vi "CoordinateConvert_WorldCartesianToShoulderOriginCartesian_Array.vi"(1 "ArmPositionIn":T1[](array[typedef]), 2 "RobotDimensions":T2) -> (0 "ArmPositionRelativeToShoulder":T1[](array[typedef]))   [LabVIEW 2018]
uses:
  TypeDefs/ConfigComponents/Config_Dimensions.ctl
  TypeDefs/ArmAbsolutePosition.ctl
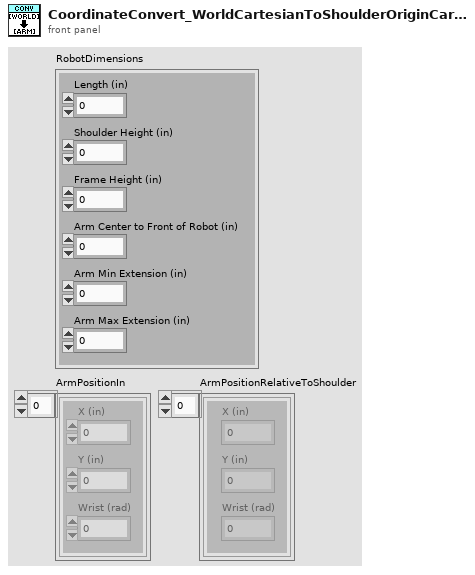
[diagram p1: front panel]
types:
  T1 = typedef "ArmAbsolutePosition.ctl" = cluster{"X (in)":dbl, "Y (in)":dbl, "Wrist (rad)":dbl}
  T2 = typedef "Config_Dimensions.ctl" = cluster{"Length (in)":dbl, "Shoulder Height (in)":dbl, "Frame Height (in)":dbl, "Arm Center to Front of Robot (in)":dbl, "Arm Min Extension (in)":dbl, "Arm Max Extension (in)":dbl}
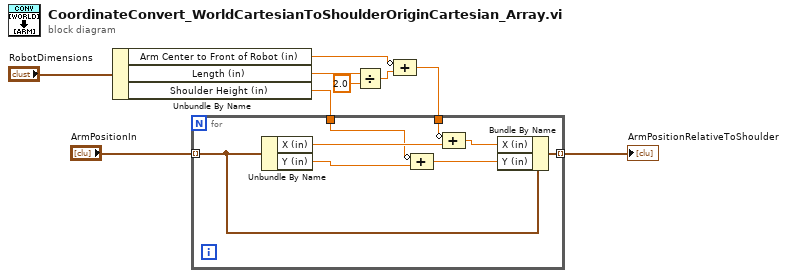
[diagram p0: block diagram]
diagram:
  n1 = Unbundle By Name("RobotDimensions") -> ("Arm Center to Front of Robot (in)"=w6:dbl, "Length (in)"=w8:dbl, "Shoulder Height (in)"=w4:dbl)
  n2 = Divide(x=w8, y=2.0) -> (x/y=w5:dbl)
  n3 = Compound Arithmetic op=ADD(invert w6, w5) -> (w3:dbl)
  n4 = for {
    tunnel: w4 -> [w10]
    tunnel: w3 -> [w16]
    tunnel: "ArmPositionIn" -> [w13] mode=indexing
    tunnel: [w12] -> w1 mode=indexing
    n5 = Unbundle By Name(w13) -> ("X (in)"=w15:dbl, "Y (in)"=w11:dbl)
    n6 = Compound Arithmetic op=ADD(invert w10, w11) -> (w17:dbl)
    n7 = Compound Arithmetic op=ADD(invert w16, w15) -> (w14:dbl)
    n8 = Bundle By Name(cluster=w13, "X (in)"=w14, "Y (in)"=w17) -> (w12:T1)
  }
  "ArmPositionRelativeToShoulder" <- w1
